vi "Introspection.vi"(8 "error in (no error)":errorcluster, 11 "ONNX Class in":refnum<class "ONNX Class.lvclass">) -> (0 "error out":errorcluster, 1 "Introspection Output":T1, 2 "Introspection Input":T1, 3 "ONNX Class out":refnum<class "ONNX Class.lvclass">)   [LabVIEW 2017, in "ONNX Class Library.lvlib" / "ONNX Class.lvclass"]
uses:
  ONNX Class.lvclass
  ONNX Class.lvclass/ONNX Class.ctl
  TypeDef/IO.ctl
  ONNX Class Library.lvlib
  TypeDef/Introspection.ctl
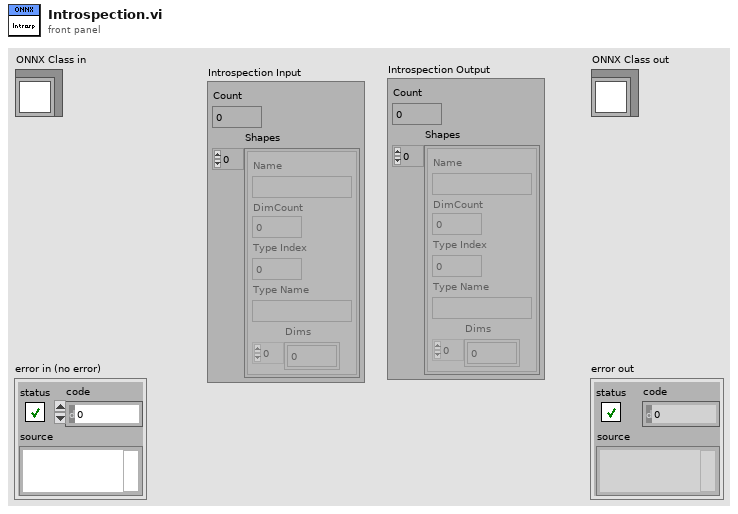
[diagram p1: front panel]
types:
  T1 = typedef "ONNX Class Library.lvlib/Introspection.ctl" = cluster{"Count":i32, "Shapes":T2[]}
  T2 = typedef "ONNX Class Library.lvlib/IO.ctl" = cluster{"Name":string, "DimCount":i32, "Type Index":i32, "Type Name":string, "Dims":i64[]}
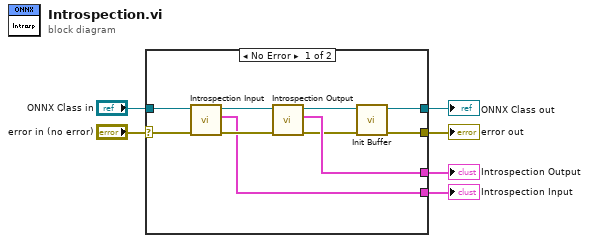
[diagram p0: block diagram]
diagram:
  n1 = case shown="No Error" "error in (no error)" {
    selector: "error in (no error)" -> [w15 w18]
    tunnel: [w7 w18] -> w5
    tunnel: [w8 w17] -> w3
    tunnel: "ONNX Class in" -> [w16 w17]
    tunnel: [w12 _] -> w2
    tunnel: [w11 _] -> w1
    frame No Error {
      n2 = call-dynamic "Introspection Input.vi"("error in (no error)"=w15, "ONNX Class in"=w16) -> ("error out"=w13:errorcluster, "Introspection Input"=w12:T1, "ONNX Class out"=w14:refnum<class "ONNX Class.lvclass">)  [unwired: 7 in]
      n3 = call-dynamic "Introspection Output.vi"("error in (no error)"=w13, "ONNX Class in"=w14) -> ("error out"=w9:errorcluster, "Introspection Output"=w11:T1, "ONNX Class out"=w10:refnum<class "ONNX Class.lvclass">)  [unwired: 7 in]
      n4 = call-dynamic "Init Buffer.vi"("error in (no error)"=w9, "ONNX Class in"=w10) -> ("error out"=w7:errorcluster, "ONNX Class out"=w8:refnum<class "ONNX Class.lvclass">)  [unwired: 8 in]
    }
    frame Error {
    }
  }
  "error out" <- w5
  "ONNX Class out" <- w3
  "Introspection Input" <- w2
  "Introspection Output" <- w1
